vi "CoreTestHarness.vi"() -> ()   [LabVIEW 2017]
uses:
  dev/Interface/Configuration.ctl
  <vilib>/rvi/Analysis/control/PID/Typedef/niFpgaPID_PIGains.ctl
  <vilib>/rvi/Analysis/control/PID/Typedef/niFpgaPID_OutputRange.ctl
  <instrlib>/_niInstr/FIFO Register Bus/v1/Host/niInstr FIFO Register Bus v1 Host.lvclass
  C:/Program Files (x86)/National Instruments/LabVIEW 2017/instr.lib/_niInstr/Instruction Framework/v1/Host/Instruction Target/niInstr Instruction Target v1 Host.lvclass
  <vilib>/FPGAPlugInAG/sbRIO-9607/niLvFpga_Open_sbRIO-9607.vi
  <vilib>/rvi/interface/common/dynamic/niFpgaDynamicAddResources.vi
  <vilib>/FPGAPlugInAG/Dynamic/niLvFpga_Reset_Dynamic.vi
  <vilib>/Utility/error.llb/Error Cluster From Error Code.vi
  <vilib>/rvi/errors/niLvFpgaAdjustHostInterfaceError.vi
  <vilib>/FPGAPlugInAG/Dynamic/niLvFpga_Run_Dynamic.vi
  <vilib>/rvi/interface/nirviOpenFPGA/nirviOpenFPGA.xnode
  dev/FPGA Bitfiles/ThreePhasePLLdev_FPGATarget_ThreePhasePLLdev_cNgKxiCEvCc.lvbitx
  dev/FPGA/ThreePhasePLL_dev.vi
  <vilib>/rvi/interface/nirviMethod/nirviMethod.xnode
  <vilib>/rvi/interface/nirviReadWriteControl/nirviReadWriteControl.xnode
  dev/Interface/ThreePhasePLLInterface.lvlib
  <vilib>/rvi/interface/Simulation/niFpgaSimulationCallBeginRW.vi
  NiFpgaLv.dll
panel:
  out "PLLTimingActual":u32
  out "ThreePhaseGenActual":u32
  out "theta error":sgl
  out "freq error":sgl
  in  "reset":bool
  out "detectedFreq":sgl
  out "Locked":bool
  in  "Configuration":T1={"PLLgains"={"proportional gain"=100.0, "integral gain"=1e-05}, "PLLrange"={"output high (Inf)"=inf, "output low (-Inf)"=0.0}, "dT"=1e-05, "expectedFreq"=376.911, "lockDuration"=3.0, "freqBoundaries"=1.0} {"PLLgains"."proportional gain" step=0.125}
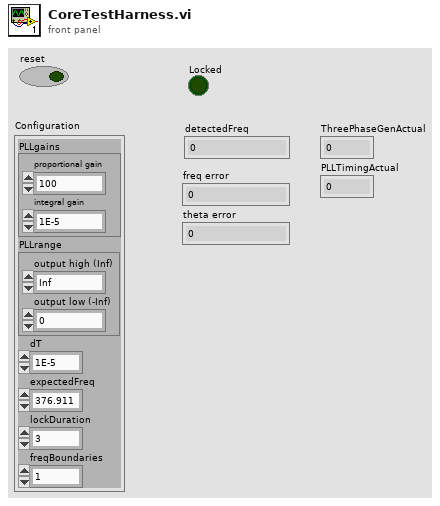
[diagram p1: front panel]
types:
  T1 = typedef "ThreePhasePLLInterface.lvlib/Configuration.ctl" = cluster{"PLLgains":T2, "PLLrange":T3, "dT":sgl, "expectedFreq":sgl, "lockDuration":sgl, "freqBoundaries":sgl}
  T2 = typedef "niFpgaPID_PIGains.ctl" = cluster{"proportional gain":sgl, "integral gain":sgl}
  T3 = typedef "niFpgaPID_OutputRange.ctl" = cluster{"output high (Inf)":sgl, "output low (-Inf)":sgl}
  T4 = typedef "ThreePhasePLLInterface.lvlib/InterfaceRef.ctl" = cluster{"instruction target":refnum<class "niInstr Instruction Target v1 Host.lvclass">, "context":refnum<class "niInstr Instruction Framework Context v1 Host.lvclass">}
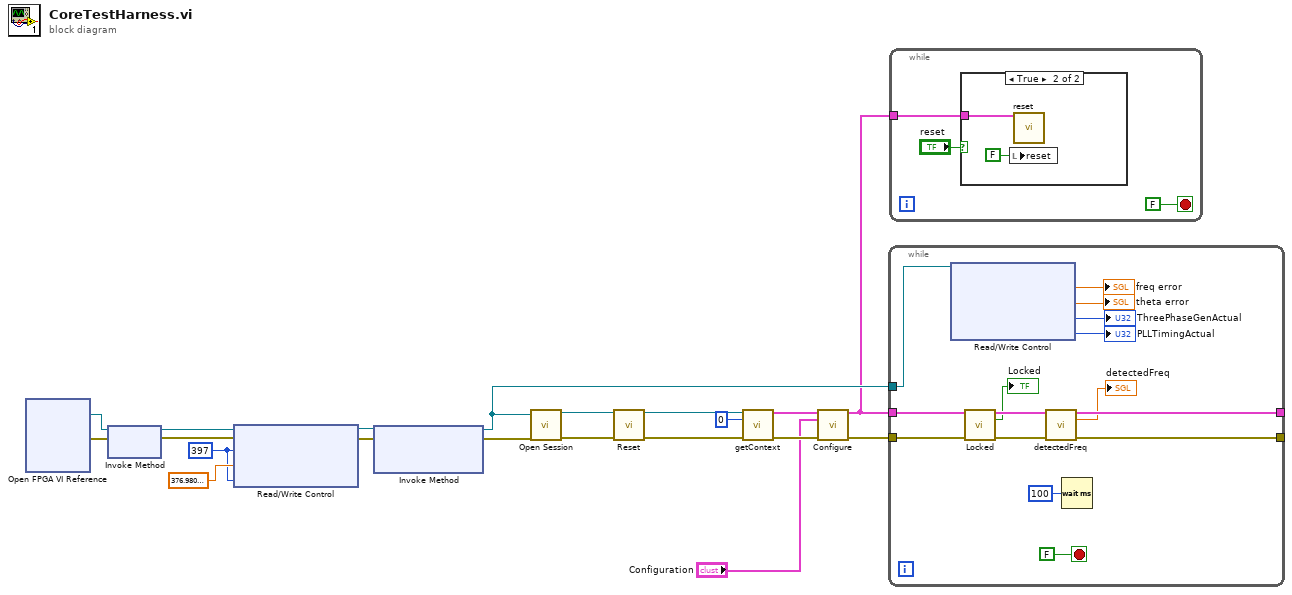
[diagram p0: block diagram]
diagram:
  w1 = u32 397 ("ThreePhaseGenTiming")
  n1 = xnode "Open FPGA VI Reference"() -> ("FPGA VI Reference Out"=w8:refnum<k20>, "error out"=w9:errorcluster)  [unwired: 2 in]
  n2 = xnode "Invoke Method"("FPGA VI Reference In"=w8, "error in"=w9) -> ("FPGA VI Reference Out"=w6:refnum<k20>, "error out"=w5:errorcluster)
  n3 = xnode "Read/Write Control"("FPGA VI Reference In"=w6, "error in"=w5, "ThreePhaseGenTiming"=w1, "GenFreqRadPerSec"=sgl 376.98, "PLL_Timing"=w1) -> ("FPGA VI Reference Out"=w4:refnum<k20>, "error out"=w3:errorcluster)
  n4 = xnode "Invoke Method"("FPGA VI Reference In"=w4, "error in"=w3) -> ("FPGA VI Reference Out"=w12:refnum<k20>, "error out"=w18:errorcluster)  [unwired: 1 in]
  n5 = call <instrlib>:"Open Session.vi"("fpga ref"=w12, "error in"=w18) -> ("session out"=w19:refnum<class "niInstr FIFO Register Bus v1 Host.lvclass">, "error out"=w20:errorcluster)  [unwired: 12 in]
  n6 = call-dynamic "Reset.vi"("session in"=w19, "error in"=w20) -> ("session out"=w17:refnum<class "niInstr FIFO Register Bus v1 Host.lvclass">, "error out"=w16:errorcluster)  [unwired: 12 in]
  n7 = call "getContext.vi"("instruction target in"=w17, "instance"=u8 0, "error in"=w16) -> ("Interface"=w14:T4, "error out"=w13:errorcluster)  [unwired: 11 in]
  n8 = call "Configure.vi"("Interface in"=w14, "Configuration"="Configuration", "error in"=w13) -> ("Interface out"=w7:T4, "error out"=w11:errorcluster)  [unwired: 11 in]
  n9 = while {
    tunnel: w12 -> [w25]
    tunnel: w11 -> [w31]
    tunnel: w7 -> [w30]
    tunnel: [w29] -> _
    tunnel: [w28] -> _
    stop <- FALSE stop-if-true
    n10 = xnode "Read/Write Control"("FPGA VI Reference In"=w25) -> ("freq error"=→"freq error":sgl, "theta error"=→"theta error":sgl, "ThreePhaseGenActual"=→"ThreePhaseGenActual":u32, "PLLTimingActual"=→"PLLTimingActual":u32)  [unwired: 1 in, 2 out]
    n11 = call "Locked.vi"("Interface in"=w30, "error in"=w31) -> ("Interface out"=w33:T4, "Locked"=→"Locked":bool, "error out"=w32:errorcluster)  [unwired: 11 in]
    n12 = call "detectedFreq.vi"("Interface in"=w33, "error in"=w32) -> ("Interface out"=w29:T4, "detectedFreq"=→"detectedFreq":sgl, "error out"=w28:errorcluster)  [unwired: 11 in]
    n13 = Wait (ms)(milliseconds to wait=u32 100) -> ()  [unwired: 1 out]
  }
  n14 = while {
    tunnel: w7 -> [w38]
    stop <- FALSE stop-if-true
    n15 = case shown="True" "reset" {
      tunnel: w38 -> [_ w39]
      frame False {
      }
      frame True {
        n16 = local write "reset"(FALSE ("reset")) -> ()
        n17 = call "reset.vi"("Interface in"=w39) -> ()  [unwired: 13 in, 2 out]
      }
    }
  }
